vi "ReadI2C.vi"(8 "error in (no error)":errorcluster, 9 "Read Data Count":i32=8, 10 "Reg Addr(Hex)":u8 format="%x", 11 "Slave Addr(Hex)":i16=80 format="%x") -> (0 "error out":errorcluster, 2 "pReadData":u8[](array[numeric]))   [LabVIEW 2024]
panel:
  in  "接口电压":i8(ring)=3 items=["0 V", "1.8 V", "2.5 V", "3.3 V"]
  in  "Channel Index":i32(ring) items=["CH0", "CH1", "CH2", "CH3", "CH4", "CH5", "CH6", "CH7"]
  in  "pConfig":T1={"ClockSpeedHz"=100000, "OwnAddr"=0, "Master"=1, "AddrBits"=7, "EnablePu"=1, "ByteIntervalUs"=0}
  in  "Device Index":i32(ring) items=["0", "1", "2", "3", "4", "5"]
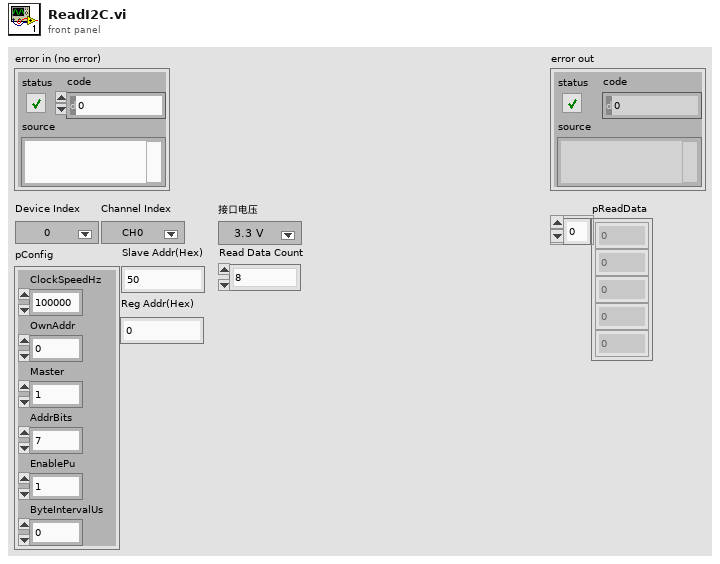
[diagram p1: front panel]
types:
  T1 = cluster{"ClockSpeedHz":u32, "OwnAddr":u16, "Master":u8, "AddrBits":u8, "EnablePu":u8, "ByteIntervalUs":u8}
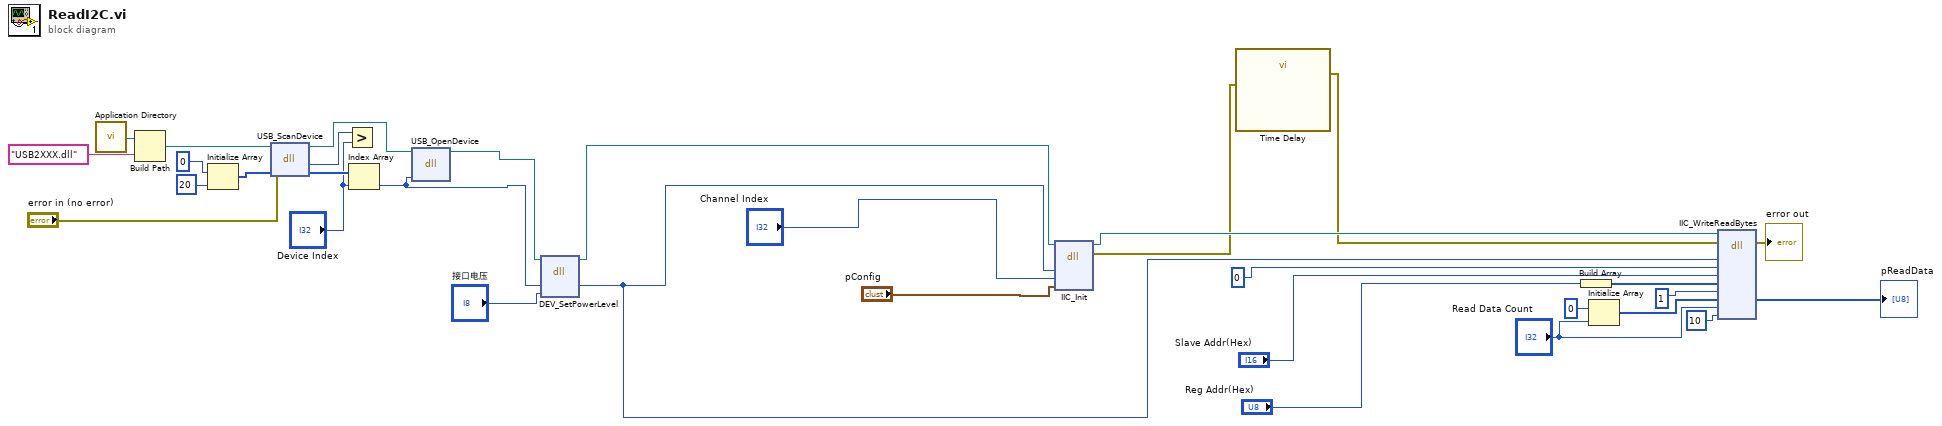
[diagram p0: block diagram]
diagram:
  n1 = call <vilib>:"Application Directory.vi"() -> ("Application Directory"=w26:path)
  n2 = Build Path(base path=w26, name or relative path="USB2XXX.dll") -> (appended path=w25:path)
  n3 = Initialize Array(0, 20 ("dimension size")) -> (w29:i32[])
  n4 = dll-call lib="D:/Project/Teststand/RFP Auto Test Sequence/Support/IIC/USB2XXX.dll" fn="USB_ScanDevice"(path in=w25, error in="error in (no error)", "pDevNum"=w29) -> (path out=w21:path, "return type"=w28:i32, "pDevNum"=w32:i32[])  [unwired: 1 in, 1 out]
  n5 = Greater?(x=w28, y="Device Index") -> ()  [unwired: 1 out]
  n6 = Index Array(array=w32, index="Device Index") -> (element=w19:i32)
  n7 = dll-call lib="D:/Project/Teststand/RFP Auto Test Sequence/Support/IIC/USB2XXX.dll" fn="USB_OpenDevice"(path in=w21, "DevIndex"=w19) -> (path out=w20:path)  [unwired: 4 in, 1 out]
  n8 = dll-call lib="D:/Project/Teststand/RFP Auto Test Sequence/Support/IIC/USB2XXX.dll" fn="DEV_SetPowerLevel"(path in=w20, "DevHandle"=w19, "PowerLevel"="接口电压") -> (path out=w18:path, "DevHandle"=w9:i32)  [unwired: 4 in, 1 out]
  n9 = dll-call lib="D:/Project/Teststand/RFP Auto Test Sequence/Support/IIC/USB2XXX.dll" fn="IIC_Init"(path in=w18, "DevIndex"=w9, "IICIndex"="Channel Index", "pConfig"="pConfig") -> (path out=w10:path, error out=w4:errorcluster)  [unwired: 6 in]
  n10 = call "Time Delay"("error in (no error)"=w4) -> ("error out"=w3:errorcluster)  [unwired: 10 in]
  n11 = Build Array("Reg Addr(Hex)") -> (w12:u8[])
  n12 = Initialize Array(u8 0 ("element"), "Read Data Count") -> (w14:u8[])
  n13 = dll-call lib="D:/Project/Teststand/RFP Auto Test Sequence/Support/IIC/USB2XXX.dll" fn="IIC_WriteReadBytes"(path in=w10, error in=w3, "DevIndex"=w9, "IICIndex"=0, "SlaveAddr"="Slave Addr(Hex)", "pWriteData"=w12, "WriteLen"=1 ("dimension size"), "pReadData"=w14, "ReadLen"="Read Data Count", "TimeOutMs"=10) -> (error out=→"error out":errorcluster, "pReadData"=→"pReadData":u8[])  [unwired: 9 in, 1 out]
